vi "Close.vi"(8 "error in (no error)":errorcluster, 9 "SubQueueIN":refnum<queue>, 10 "MainQueueIN":refnum<queue>, 11 "Data Value Reference IN":refnum<data-value>) -> (0 "error out":errorcluster, 3 "Data Value Reference out":refnum<data-value>)   [LabVIEW 2013]
uses:
  Control/SystemCommand.ctl
  Control/SystemData.ctl
  Control/SignalType.ctl
  Control/SubDaqCommand.ctl
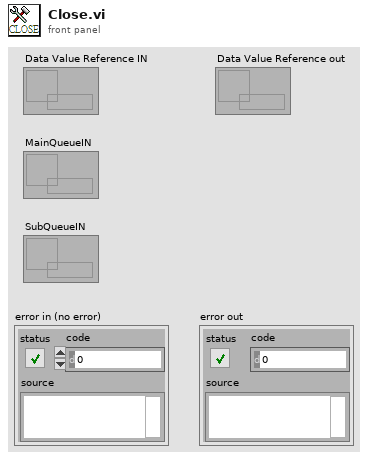
[diagram p1: front panel]
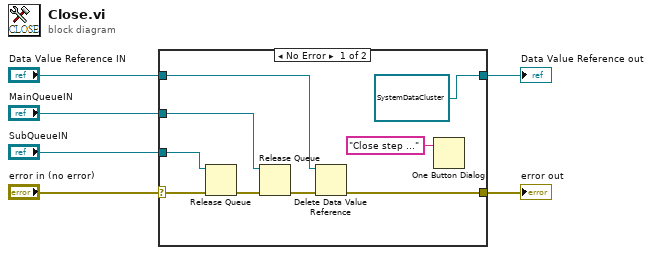
[diagram p0: block diagram]
diagram:
  n1 = case shown="No Error" "error in (no error)" {
    selector: "error in (no error)" -> [w7 w16]
    tunnel: "Data Value Reference IN" -> [w12 w17]
    tunnel: [refnum<data-value> refnum ("Data Value Reference IN") w17] -> w3
    tunnel: [w10 w16] -> w5
    tunnel: "MainQueueIN" -> [w13 _]
    tunnel: "SubQueueIN" -> [w8 _]
    frame No Error {
      n2 = Release Queue(queue=w8, error in (no error)=w7) -> (error out=w9:errorcluster)  [unwired: 1 in, 2 out]
      n3 = Release Queue(queue=w13, error in (no error)=w9) -> (error out=w14:errorcluster)  [unwired: 1 in, 2 out]
      n4 = Delete Data Value Reference(data value reference=w12, error in=w14) -> (error out=w10:errorcluster)  [unwired: 1 out]
      n5 = One Button Dialog(message="Close step ...") -> ()  [unwired: 1 in, 1 out]
    }
    frame Error {
    }
  }
  "error out" <- w5
  "Data Value Reference out" <- w3
